vi "NonReentrantMeasurement_MultipleMeasureCalls_ExecuteInSequence.vi"(8 "error in":errorcluster, 11 "run service vi":refnum<vi>) -> (0 "error out":errorcluster, 1 "result":string, 2 "pass":bool)   [LabVIEW 2021]
uses:
  Runtime/Measurements/Helpers/TypeDefs/Measurement Server User Settings.ctl
  Runtime/Measurements/Helpers/TypeDefs/Stop Server User Event.ctl
  Runtime/Measurements/Helpers/TypeDefs/Measurement Service Version.ctl
  Continuous Counting Client/controls/Measurement Configuration.ctl
  Runtime/Measurements/NI Measurement Plug-In SDK.lvlib
  Continuous Counting Client/Continuous Counting Client.lvlib
  MeasurementServerTests.lvlib
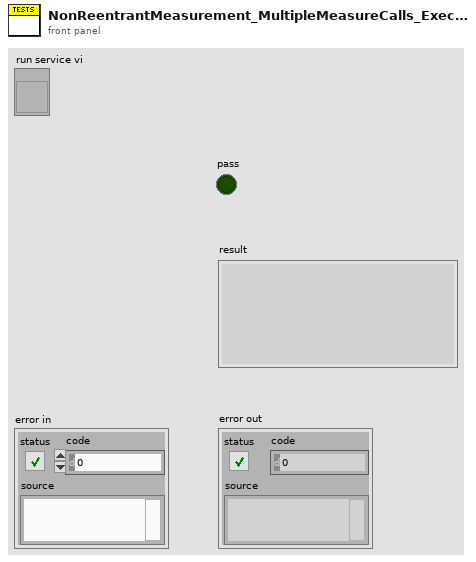
[diagram p1: front panel]
types:
  T1 = typedef "NI Measurement Plug-In SDK.lvlib/Measurement Service Version.ctl" = enum16{"V1", "V2"}
  T2 = typedef "NI Measurement Plug-In SDK.lvlib/Measurement Server User Settings.ctl" = cluster{"stop server":T3, "measurement service versions":T1[]}
  T3 = typedef "NI Measurement Plug-In SDK.lvlib/Stop Server User Event.ctl" = refnum<user-event>
  T4 = typedef "grpc-lvsupport-release.lvlib/grpcId.ctl" = u64
  T5 = typedef "MeasurementServerTests.lvlib/Measurement Service Tests.lvlib/Continuous Counting Client.lvlib/Measurement Configuration.ctl" = cluster{"ms update interval":u32}
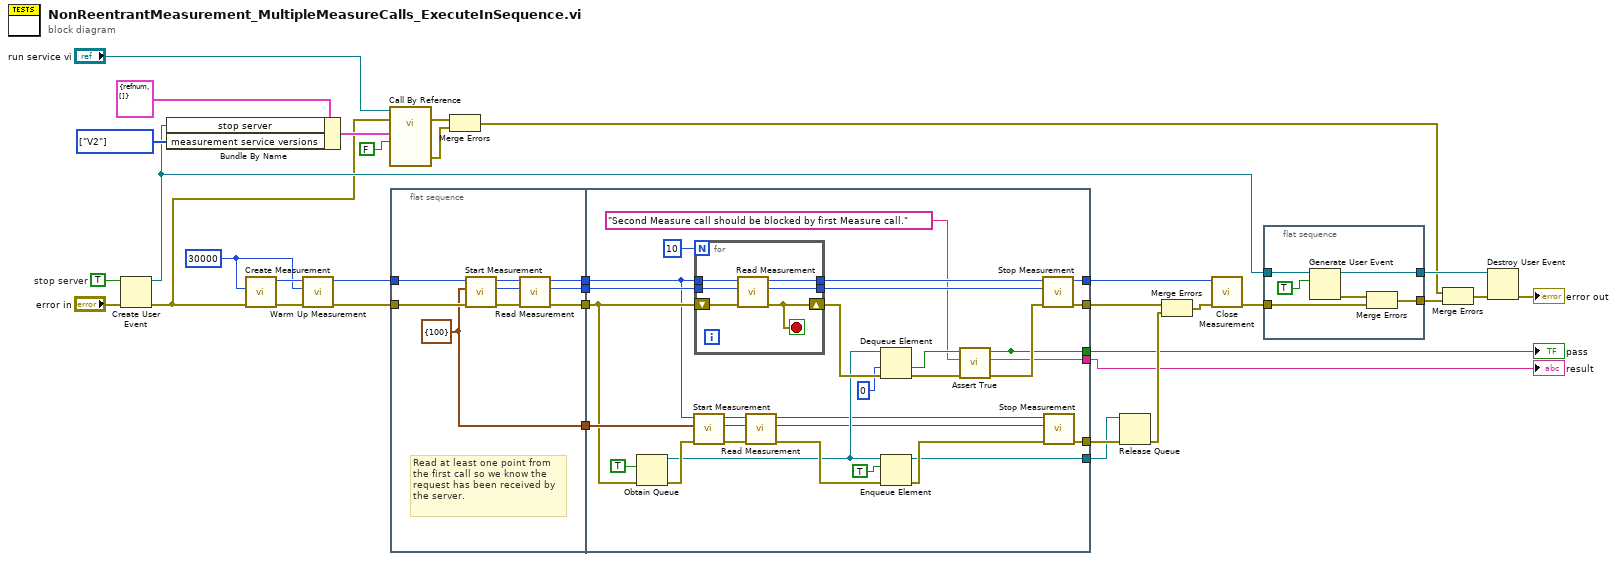
[diagram p0: block diagram]
diagram:
  w12 = 30000 ("ms timeout")
  w32 = TRUE  # stop server
  w33 = T1[] [enum."V2"] items=["V1", "V2"] ("measurement service versions")
  n1 = Create User Event(user event datatype=w32, error in="error in") -> (user event=w29:refnum<user-event>, error out=w4:errorcluster)
  n2 = Bundle By Name(cluster=T2 {"stop server"=refnum, "measurement service versions"=[]} ("server settings"), "stop server"=w29, "measurement service versions"=w33) -> (w6:T2)
  n3 = call "Create Measurement.vi"("error in"=w4, "ms timeout"=w12) -> ("error out"=w16:errorcluster, "gRPCid out"=w13:T4)  [unwired: 8 in]
  n4 = call "Warm Up Measurement.vi"("error in"=w16, "timeout (ms)"=w12, "gRPC ID"=w13) -> ("error out"=w15:errorcluster, "gRPC ID out"=w14:T4)  [unwired: 7 in]
  n5 = call-by-ref "?"(reference="run service vi", error in=w4, "reentrant"=FALSE, "server settings"=w6) -> (error out=w3:errorcluster, 0:"error out"=w2:errorcluster)  [unwired: 9 in, 1 out]
  n6 = flat-sequence {
    tunnel: w15 -> [w43]
    tunnel: w14 -> [w42]
    tunnel: [w39] -> w27
    tunnel: [w38] -> w26
    tunnel: [w35] -> w25
    tunnel: [w36] -> w24
    tunnel: [w67] -> w21
    tunnel: w27 -> [w64]
    tunnel: w26 -> [w44]
    tunnel: w25 -> [w73]
    tunnel: w24 -> [w68]
    tunnel: [w53] -> w23
    tunnel: [w48] -> w22
    tunnel: [w47] -> w19
    tunnel: [w45] -> _
    tunnel: [w46] -> w18
    tunnel: [w45] -> w17
    frame #0 {
      w36 = T5 {"ms update interval"=100} ("measurement configuration")
      # "Read at least one point from\nthe first call so we know the\nrequest has been received by\nthe server."
      n7 = call "Start Measurement.vi"("error in"=w43, "measurement configuration"=w36, "gRPCid in"=w42) -> ("error out"=w40:errorcluster, "call id"=w37:T4, "gRPCid out"=w41:T4)  [unwired: 6 in]
      n8 = call "Read Measurement.vi"("error in"=w40, "call id in"=w37, "gRPCid in"=w41) -> ("error out"=w39:errorcluster, "call id out"=w35:T4, "gRPCid out"=w38:T4)  [unwired: 4 in, 2 out]
    }
    frame #1 {
      n9 = Obtain Queue(element data type=TRUE, error in (no error)=w64) -> (queue out=w58:refnum<queue>, error out=w62:errorcluster)  [unwired: 3 in, 1 out]
      n10 = call "Start Measurement.vi"("error in"=w62, "measurement configuration"=w68, "gRPCid in"=w44) -> ("error out"=w71:errorcluster, "call id"=w69:T4, "gRPCid out"=w70:T4)  [unwired: 6 in]
      n11 = for {
        N: 10 -> [_]
        shift-right: [w75] -> w59
        shift-left: w64 -> [w79]
        tunnel: w44 -> [w78]
        tunnel: w73 -> [w77]
        tunnel: [w76] -> w66
        tunnel: [w74] -> w65
        stop <- w75 stop-if-true
        n12 = call "Read Measurement.vi"("error in"=w79, "call id in"=w77, "gRPCid in"=w78) -> ("error out"=w75:errorcluster, "call id out"=w74:T4, "gRPCid out"=w76:T4)  [unwired: 4 in, 2 out]
      }
      n13 = call "Read Measurement.vi"("error in"=w71, "call id in"=w69, "gRPCid in"=w70) -> ("error out"=w61:errorcluster, "call id out"=w55:T4, "gRPCid out"=w56:T4)  [unwired: 4 in, 2 out]
      n14 = Dequeue Element(queue=w58, timeout in ms (-1)=0, error in (no error)=w59) -> (timed out?=w50:bool, error out=w52:errorcluster)  [unwired: 2 out]
      n15 = Enqueue Element(queue=w58, element=TRUE, error in (no error)=w61) -> (queue out=w48:refnum<queue>, error out=w54:errorcluster)  [unwired: 1 in, 1 out]
      n16 = call "Assert True.vi"("error in"=w52, "failure message"="Second Measure call should be blocked by first Measure call.", "condition"=w50) -> ("error out"=w51:errorcluster, "message"=w46:string, "pass"=w45:bool)  [unwired: 6 in]
      n17 = call "Stop Measurement.vi"("error in"=w51, "call id"=w65, "gRPCid in"=w66) -> ("error out"=w67:errorcluster, "gRPCid out"=w47:T4)  [unwired: 7 in]
      n18 = call "Stop Measurement.vi"("error in"=w54, "call id"=w55, "gRPCid in"=w56) -> ("error out"=w53:errorcluster)  [unwired: 7 in, 1 out]
    }
  }
  n19 = Merge Errors(w3, w2) -> (w1:errorcluster)
  n20 = Release Queue(queue=w22, error in (no error)=w23) -> (error out=w20:errorcluster)  [unwired: 1 in, 2 out]
  n21 = Merge Errors(w21, w20) -> (w30:errorcluster)
  n22 = call "Close Measurement.vi"("error in"=w30, "gRPCid in"=w19) -> ("error out"=w28:errorcluster)  [unwired: 9 in]
  n23 = flat-sequence {
    tunnel: w29 -> [w84]
    tunnel: [w83] -> w9
    tunnel: [w82] -> w11
    tunnel: w28 -> [w81]
    frame #0 {
      n24 = Generate User Event(user event=w84, event data cluster=TRUE ("event data")) -> (user event out=w83:refnum<user-event>, error out=w85:errorcluster)  [unwired: 2 in]
      n25 = Merge Errors(w85, w81) -> (w82:errorcluster)
    }
  }
  n26 = Merge Errors(w1, w11) -> (w10:errorcluster)
  n27 = Destroy User Event(user event=w9, error in=w10) -> (error out=→"error out":errorcluster)
  "pass" <- w17
  "result" <- w18
